vi "Read MarkerSkill.lvclass.vi"(8 "error in (no error)":errorcluster, 11 "Skillbook in":refnum<class "Skillbook.lvclass">) -> (0 "error out":errorcluster, 2 "MarkerSkill.lvclass":refnum<class "MarkerSkill.lvclass">, 3 "Skillbook out":refnum<class "Skillbook.lvclass">)   [LabVIEW 2018, in "Skillbook.lvclass"]
uses:
  Skillbook.lvclass
  MarkerSkill_class/MarkerSkill.lvclass
  Skillbook.lvclass/Skillbook.ctl
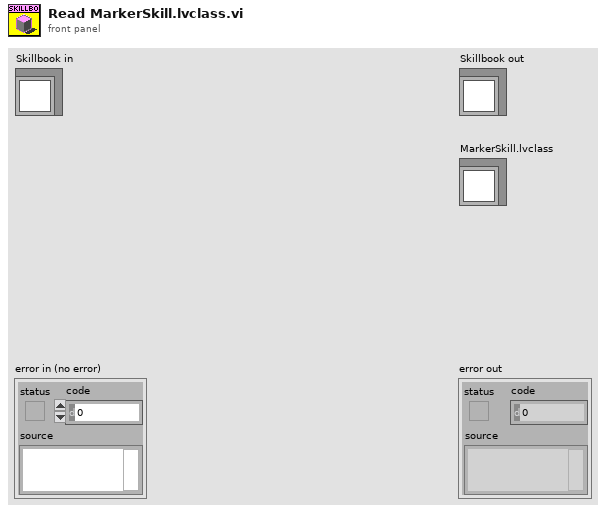
[diagram p1: front panel]
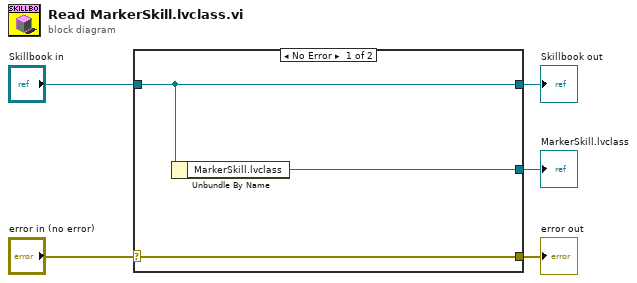
[diagram p0: block diagram]
diagram:
  n1 = case shown="No Error" "error in (no error)" {
    selector: "error in (no error)" -> [w8 w9]
    tunnel: [w8 w9] -> w4
    tunnel: [w7 w10] -> w2
    tunnel: "Skillbook in" -> [w7 w10]
    tunnel: [w6 _] -> w1
    frame No Error {
      n2 = Unbundle By Name(w7) -> ("MarkerSkill.lvclass"=w6:refnum<class "MarkerSkill.lvclass">)
    }
    frame Error {
    }
  }
  "error out" <- w4
  "Skillbook out" <- w2
  "MarkerSkill.lvclass" <- w1
